vi "ColorSensor Controller Interactive Check.vi"(8 "Interactive Command in":T1, 9 "Default Command":T1, 11 "Buttons":cluster{"Execute Cmd":bool, "Abort Cmd":bool}) -> (1 "Interactive Command out":T1, 2 "Trace String":string, 3 "Schedule":bool)   [LabVIEW 2019]
doc: "Check the Execute and Abort buttons and choose the data and trace string."
uses:
  ColorSensor Setpoints.ctl
  ColorSensor Operations.ctl
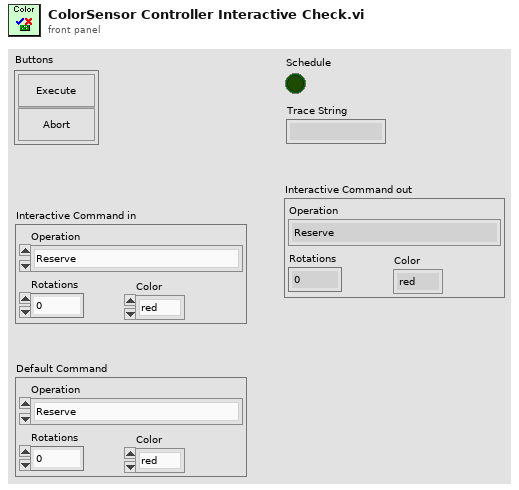
[diagram p1: front panel]
types:
  T1 = typedef "ColorSensor Setpoints.ctl" = cluster{"Operation":T2, "Rotations":dbl, "Color":enum16{"red", "blue", "yellow", "green"}}
  T2 = typedef "ColorSensor Operations.ctl" = enum16{"Reserve", "spin_to_color", "Read Current", "ColorSpin", "Immediate"}
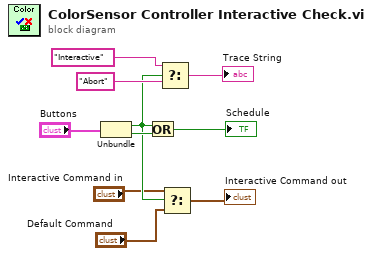
[diagram p0: block diagram]
diagram:
  n1 = Unbundle("Buttons") -> ("Execute Cmd"=w6:bool, "Abort Cmd"=w7:bool)
  n2 = Or(x=w6, y=w7) -> (x .or. y?=→"Schedule":bool)
  n3 = Select(t="Interactive", s=w6, f="Abort") -> (s? t:f=→"Trace String":string)
  n4 = Select(t="Interactive Command in", s=w6, f="Default Command") -> (s? t:f=→"Interactive Command out":T1)
